vi "PH_USB600x_AnalogReader.read Database.vi"(0 "i ref in":refnum<vi>, 5 "error in (no error)":errorcluster) -> (14 "i ref out":refnum<vi>, 16 "Port":string, 19 "error out":errorcluster)   [LabVIEW 2014, in "PH_USB600x_AnalogReader.lvlib"]
doc: "Reads the database and inizialises the physical channels of the device\n\nLicense Agreement for the BaseProcess class:\n\nCopyright (C)\nGesellschaft für Schwerionenforschung, GSI\nPlanckstr. 1\n64291 Darmstadt\nGermany\n\nContact: D.Beck@gsi.de \n\nThis program is free software; you can redistribute it and/or modify it under the terms of the \nGNU General Public License as published by the Free Software Foundation; either version 2 of the license, or (at your option) any later version.\n\nThis program is distributed in the hope that it will be useful, but WITHOUT ANY WARRANTY; without even the implied warranty of MERCHANTABILITY or FITNESS FOR A PARTICULAR PURPOSE. See the GNU General License for more details (http://www.gnu.org).\n\nGesellschaft für Schwerionenforschung, GSI\nPlanckstr. 1, 64291 Darmstadt, Germany\nFor all questions and ideas contact: M.Richter@gsi.de, H.Brand@gsi.de or D.Beck@gsi.de.\nLast update: 25-SEP-2002"
uses:
  PH_USB600x_AnalogReader.lvlib
  PH_Basics/PH_StatusHandler/PH_StatusHandler.Status.ctl
  <vilib>/DAQmx/create/channels.llb/DAQmx Create Channel (AI-Voltage-Basic).vi
  CS_Core/CSSystem/CSSystemLib/CSSystemLib.lvlib
  PH_Basics/PH_StatusHandler/PH_StatusHandler.lvlib
  PH_Basics/PH_Common/PH_Common.lvlib
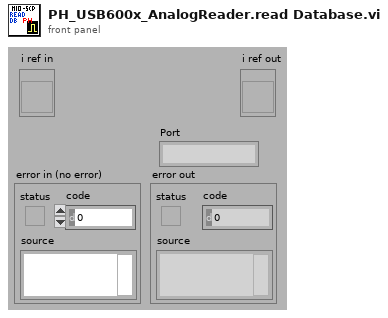
[diagram p1: front panel]
types:
  T1 = typedef "PH_USB600x_AnalogReader.lvlib/PH_USB600x_AnalogReader.i attribute.ctl" = cluster{"GUI Refs":cluster{"Delete":refnum<vi>, "Status":refnum<vi>, "Timeout":refnum<vi>, "Acquire Waveform":refnum<vi>, "Timing":refnum<vi>, "Graph":refnum<vi>, "Prdc Interval":refnum<vi>, "Formula":refnum<vi>}, "Device Settings":cluster{"AIChannel":refnum<k21>, "channelName":string, "Status":T2}, "Timing":T3, "Prdc Interval":dbl, "Lin Scaling":T4, "Data":cluster{"t0":timestamp, dbl}[]}
  T2 = typedef "PH_StatusHandler.lvlib/PH_StatusHandler.Status.ctl" = i16
  T3 = typedef "PH_USB600x_AnalogReader.lvlib/PH_USB600x_AnalogReader.Timing.ctl" = cluster{"Samples per Channel":i32, "Rate":dbl}
  T4 = typedef "PH_USB600x_AnalogReader.lvlib/PH_USB600x_AnalogReader.Lin Scaling.ctl" = cluster{"Slope [Unit/V]":dbl, "Offset [Unit]":dbl, "Y-Unit":string, "Y-Label":string}
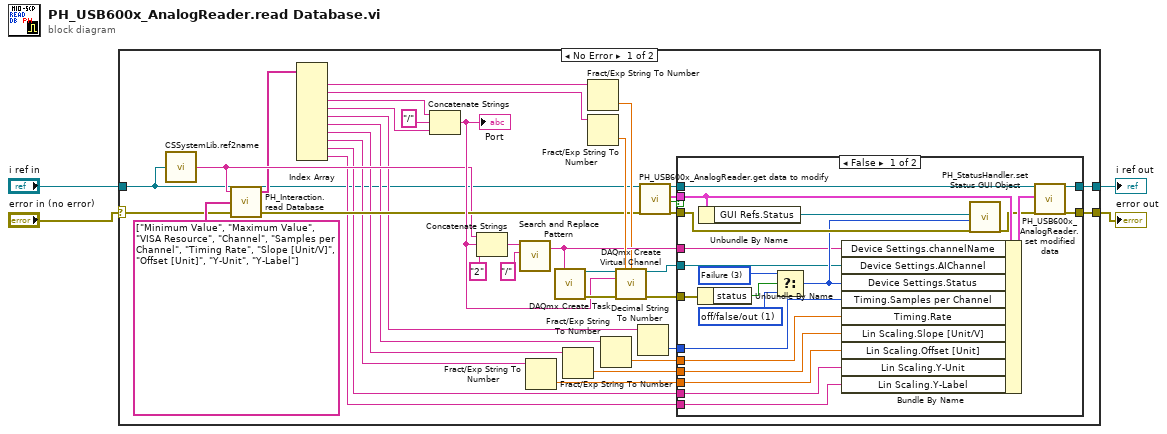
[diagram p0: block diagram]
diagram:
  n1 = case shown="No Error" "error in (no error)" {
    selector: "error in (no error)" -> [w5 w66]
    tunnel: "i ref in" -> [w6 w67]
    tunnel: [w36 w66] -> w3
    tunnel: [w37 w67] -> w2
    frame No Error {
      n2 = call "CSSystemLib.ref2name.vi"("obj refnum"=w6) -> ("name"=w19:string)
      n3 = call "PH_Interaction.read Database.vi"("error in (no error)"=w5, "Strings to search for"=string[] ["Minimum Value", "Maximum Value", "VISA Resource", "Channel", "Samples per Channel", "Timing Rate", "Slope [Unit/V]", "Offset [Unit]", "Y-Unit", "Y-Label"], "DB Entry to read"=w19) -> ("error out"=w20:errorcluster, "Values"=w17:string[])  [unwired: 1 in]
      n4 = Index Array(array=w17) -> (element #1=w14:string, element #2=w13:string, element #3=w16:string, element #4=w15:string, element #5=w11:string, element #6=w12:string, element #7=w10:string, element #8=w9:string, element #9=w8:string, element #10=w7:string)  [unwired: 10 in]
      n5 = Concatenate Strings(w16, "/" ("string"), w15) -> (w21:string)
      "Port" <- w21
      n6 = Concatenate Strings(w19, w21, "2") -> (w33:string)
      n7 = call <vilib>:"Search and Replace Pattern.vi"("string"=w33, "regular expression (\"\")"="/" ("regular expression (\"\")")) -> ("result string"=w28:string)  [unwired: 3 in, 1 out]
      n8 = Fract/Exp String To Number(string=w9) -> (number=w23:dbl)  [unwired: 3 in, 1 out]
      n9 = call <vilib>:"DAQmx Create Task.vi"("new task name"=w28) -> ("task out"=w35:refnum<k21>, "error out"=w34:errorcluster)  [unwired: 13 in]
      n10 = Fract/Exp String To Number(string=w10) -> (number=w24:dbl)  [unwired: 3 in, 1 out]
      n11 = Fract/Exp String To Number(string=w14) -> (number=w22:dbl)  [unwired: 3 in, 1 out]
      n12 = Fract/Exp String To Number(string=w13) -> (number=w30:dbl)  [unwired: 3 in, 1 out]
      n13 = Fract/Exp String To Number(string=w12) -> (number=w25:dbl)  [unwired: 3 in, 1 out]
      n14 = call-poly <vilib>:"DAQmx Create Virtual Channel.vi"("task in"=w35, "maximum value"=w30, "minimum value"=w22, "physical channels"=w21, "error in"=w34) -> ("task out"=w29:refnum<k21>, "error out"=w27:errorcluster)  [unwired: 9 in]
      n15 = Decimal String To Number(string=w11) -> (number=w26:i32)  [unwired: 2 in, 1 out]
      n16 = call "PH_USB600x_AnalogReader.get data to modify.vi"("i ref in"=w6, "error in (no error)"=w20) -> ("i ref out"=w39:refnum<vi>, "i attribute"=w41:T1, "timed out"=w38:bool, "error out"=w40:errorcluster)  [unwired: 14 in]
      n17 = case shown="False" w38 {
        tunnel: [w63 w65] -> w37
        tunnel: w39 -> [w61 w65]
        tunnel: [w62 w64] -> w36
        tunnel: w40 -> [w56 w64]
        tunnel: w41 -> [w58 _]
        tunnel: w28 -> [w44 _]
        tunnel: w29 -> [w45 _]
        tunnel: w27 -> [w59 _]
        tunnel: w26 -> [w50 _]
        tunnel: w25 -> [w49 _]
        tunnel: w24 -> [w48 _]
        tunnel: w23 -> [w47 _]
        tunnel: w8 -> [w46 _]
        tunnel: w7 -> [w43 _]
        frame False {
          w52 = T2 1 items=["no info", "off/false/out", "on/true/in", "Failure", "Alarm", "Status 1", "Status 2", "Status 3"] ("Device Settings.Status")
          w53 = T2 3 items=["no info", "off/false/out", "on/true/in", "Failure", "Alarm", "Status 1", "Status 2", "Status 3"] ("Device Settings.Status")
          n18 = Unbundle By Name(w59) -> ("status"=w54:bool)
          n19 = Unbundle By Name(w58) -> ("GUI Refs.Status"=w57:refnum<vi>)
          n20 = Select(t=w53, s=w54, f=w52) -> (s? t:f=w51:T2)
          n21 = Bundle By Name(cluster=w58, "Device Settings.channelName"=w44, "Device Settings.AIChannel"=w45, "Device Settings.Status"=w51, "Timing.Samples per Channel"=w50, "Timing.Rate"=w49, "Lin Scaling.Slope [Unit/V]"=w48, "Lin Scaling.Offset [Unit]"=w47, "Lin Scaling.Y-Unit"=w46, "Lin Scaling.Y-Label"=w43) -> (w60:T1)
          n22 = call "PH_StatusHandler.set Status GUI Object.vi"("PH Status Ref"=w57, "Value"=w51, "error in (no error)"=w56) -> ("error out"=w55:errorcluster)  [unwired: 16 in]
          n23 = call "PH_USB600x_AnalogReader.set modified data.vi"("i ref in"=w61, "i attribute"=w60, "error in (no error)"=w55) -> ("i ref out"=w63:refnum<vi>, "error out"=w62:errorcluster)  [unwired: 15 in]
        }
        frame True {
        }
      }
    }
    frame Error {
    }
  }
  "error out" <- w3
  "i ref out" <- w2
